vi "LoadGainCorrectionImages.vi"(8 "Pixel calibration":T1, 10 "MeasureConfig":T3={"Bead locations"=[{"X"=0, "Y"=0}], "ROI"=200, "Experiment base path"=path "", "Image output subdir"="images", "Output mode"=enum."None", "Traces output subdir"="traces", "QTrk Settings"={"Image width"=150, "Image height"=150, "Number of threads (CPU based)"=-1, "CUDA Device"=-2, "COM Background correction factor"=0.0, "ZLUT MinRadius"=8.0, "ZLUT Radial sample density"=5.0, "ZLUT Angular sample density"=2.0, "ZLUT ROI Coverage"=0.7, "QI Iterations"=1, "QI MinRadius"=2.0, "QI Radial sample density"=5.0, "QI Angular sample density"=2.0, "QI ROI Coverage"=0.7, "QI Angular Step \nIteration Factor"=0.8, "XCOR Profile Length"=1, "XCOR Profile Width"=128, "XCOR Iterations"=32, "Gaussian 2D Fit Iterations"=2, "Gaussian 2D Sigma (pixels)"=3.0, "Downsample"=0}, "Tracking Config"={"Number of steps"=0, "ZLUT stepsize (um)"=0.0, "Z correction factor"=0.0, "Start piezo Z (um)"=0.0, "Pixel size (nm)"=0.0, "2D Localization Type"=enum."Quadrant Interpolation", "Z Command (None)"=enum."Nothing", "Z Piezo scale"=FALSE, "ZLUT Building\nimages per frame"=1}, "Experiment Name"="", "Program"={"Commands"=[], "Motor Axis accuracy conditions"={"Magnet Z"=0.0, "Magnet rotation"=0.0, "Camera"={"X"=0.0, "Y"=0.0}, "Piezo XY"={"X"=0.0, "Y"=0.0}, "Piezo Z"=0.0, "Coil XY"={"X"=0.0, "Y"=0.0}}, "Axis flags"={"Magnet Z"=FALSE, "Magnet rotation"=FALSE, "Camera"={"X"=FALSE, "Y"=FALSE}, "Piezo XY"={"X"=FALSE, "Y"=FALSE}, "Piezo Z"=FALSE, "Coil XY"={"X"=FALSE, "Y"=FALSE}}}, "ZLUT"=[], "Camera settings"={"Framerate (Hz)"=60, "Exposure time (us)"=5000, "Image size"={"Width"=1280, "Height"=1024}, "Number of buffers"=30}, "Experiment Script"="", "Max frames in memory"=10000, "Save traces as binary"=FALSE, "Pixel Calibration Gain Image"="camera_calib_gain.bin", "Pixel Calibration Offset Image"="camera_calib_offset.bin", "Use pixel calibration images"=FALSE, "Internal camera settings"="", "Trace write interval"=100} {"QTrk Settings"."QI ROI Coverage" format="%_2g"; "QTrk Settings"."QI MinRadius" format="%.2f"; "QTrk Settings"."QI Angular sample density" format="%.3f"; "QTrk Settings"."QI Radial sample density" format="%.2f"; "QTrk Settings"."ZLUT Radial sample density" format="%.2f"; "QTrk Settings"."ZLUT MinRadius" format="%.2f"}, 11 "QTrk Instance in":T17) -> (0 "Pixel calibration(out)":T1, 3 "QTrk Instance out":T17)   [LabVIEW 2011]
uses:
  qtrk/QTrkLVBinding/QTrkInstance.ctl
  Typedefs/MeasureConfigType.ctl
  Typedefs/MeasureConfigOutputMode.ctl
  qtrk/QTrkLVBinding/QTrkSettings.ctl
  Typedefs/TrackingConfigType.ctl
  qtrk/QTrkLVBinding/QTrkLocalizationType.ctl
  qtrk/QTrkLVBinding/QTrkZCommandType.ctl
  ExperimentProgram/ExperimentProgramType.ctl
  ExperimentProgram/ExProgCommandType.ctl
  ExperimentProgram/ExProgCommandEnumType.ctl
  Motors/MotorAxisEnum.ctl
  Motors/MotorPosType.ctl
  Typedefs/XYf.ctl
  Motors/MotorPosFlagsType.ctl
  Camera/GenericCameraConfigType.ctl
  Camera/PixelCalibrationDataType.ctl
  <vilib>/vision/Image Controls.llb/IMAQ Image.ctl
panel:
  # "(used for commands with string parameters)"
  # "-2: Use all devices\n-1: Use best device"
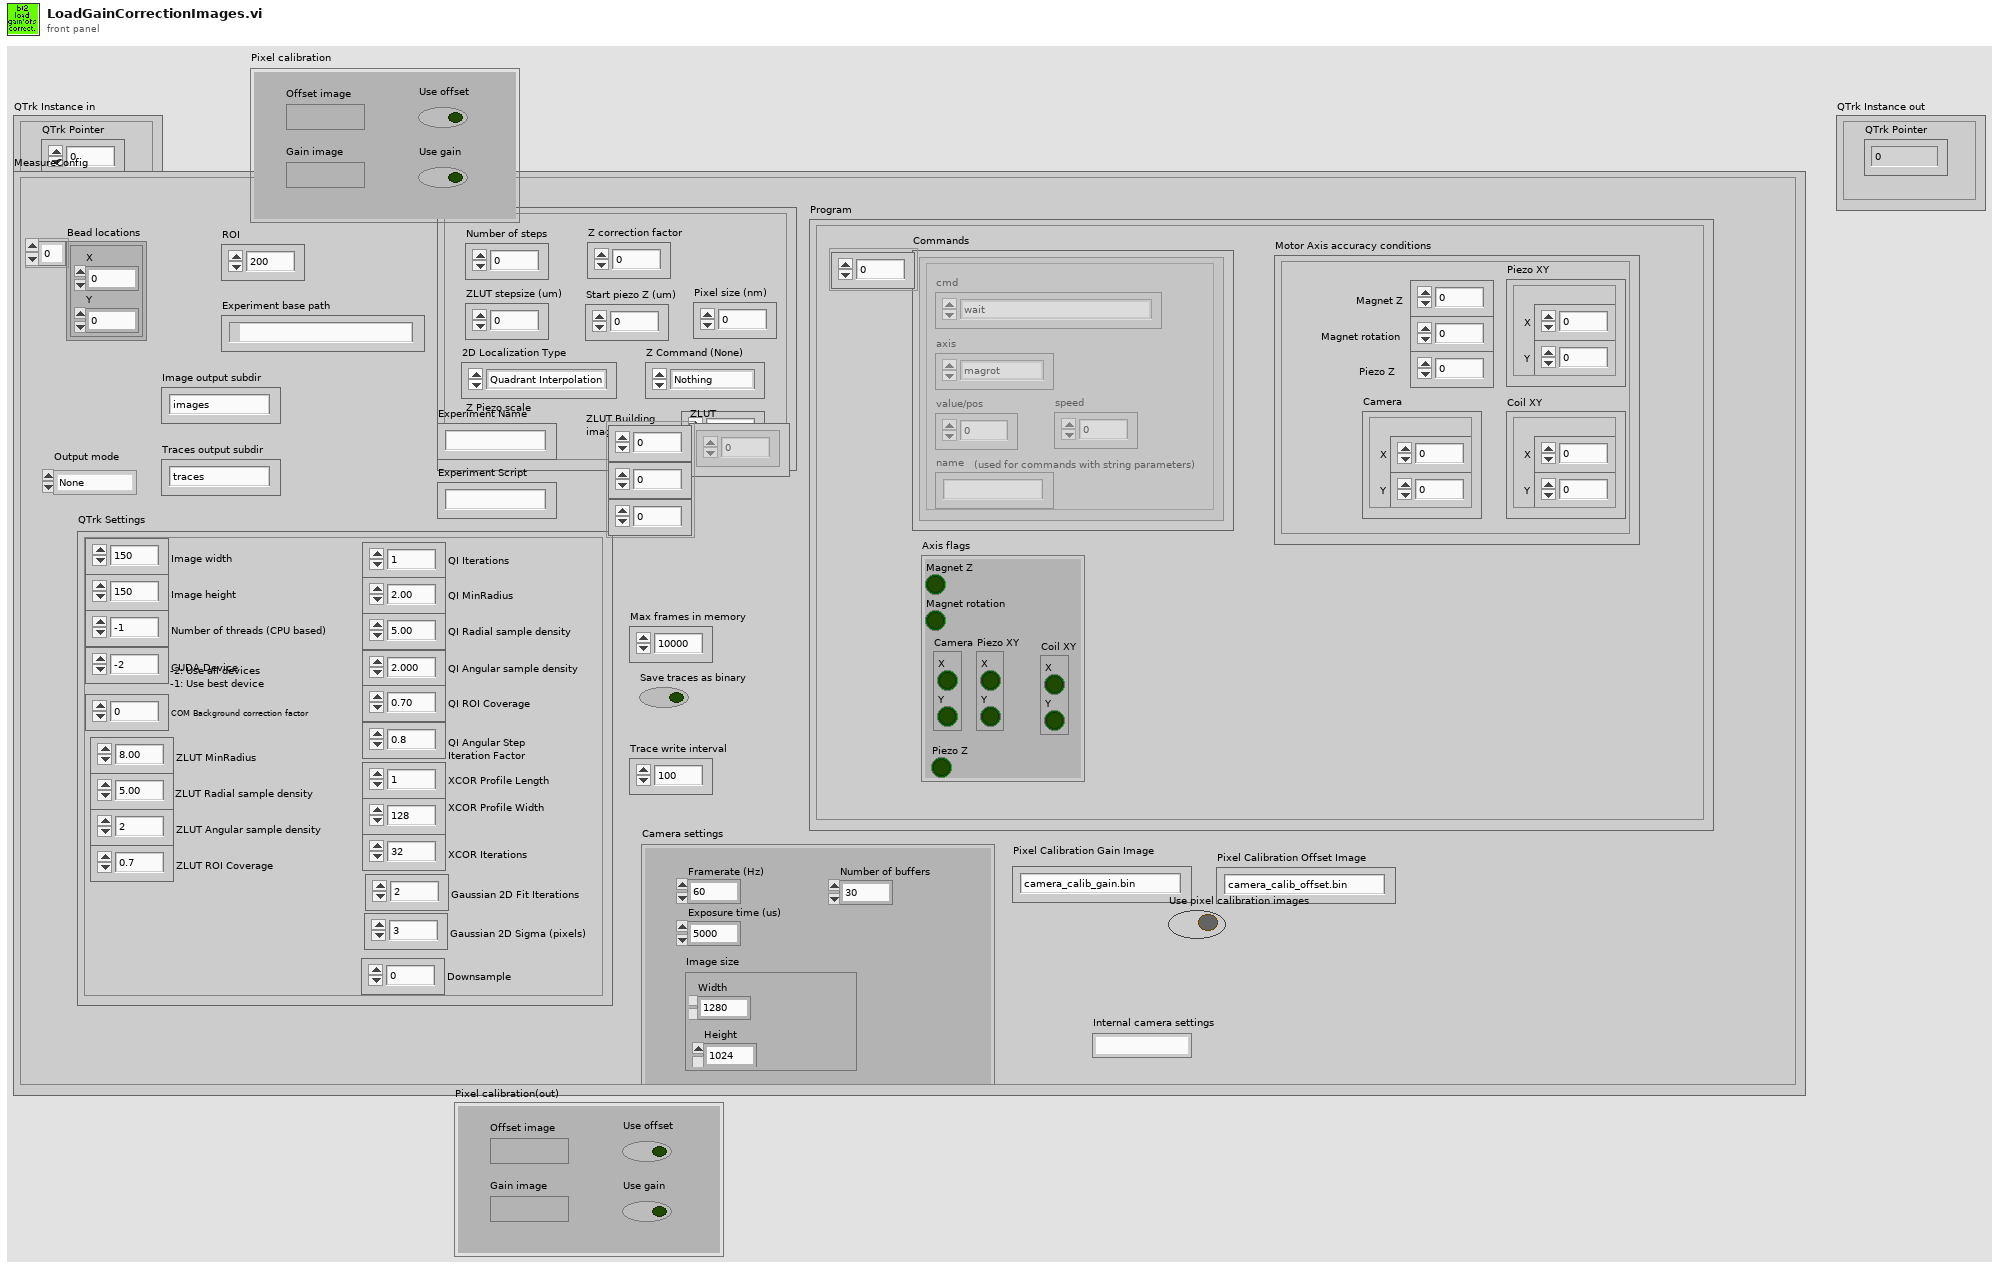
[diagram p1: front panel]
types:
  T1 = typedef "PixelCalibrationDataType.ctl" = cluster{"Offset image":T2, "Gain image":T2, "Use offset":bool, "Use gain":bool}
  T2 = typedef "IMAQ Image.ctl" = refnum<image>
  T3 = typedef "MeasureConfigType.ctl" = cluster{"Bead locations":cluster{"X":i32, "Y":i32}[], "ROI":i32, "Experiment base path":path, "Image output subdir":string, "Output mode":T4, "Traces output subdir":string, "QTrk Settings":T5, "Tracking Config":T6, "Experiment Name":string, "Program":T9, "ZLUT":sgl[][][], "Camera settings":T16, "Experiment Script":string, "Max frames in memory":i32, "Save traces as binary":bool, "Pixel Calibration Gain Image":string, "Pixel Calibration Offset Image":string, "Use pixel calibration images":bool, "Internal camera settings":string, "Trace write interval":i32}
  T4 = typedef "MeasureConfigOutputMode.ctl" = enum16{"None", "Track", "SaveImages"}
  T5 = typedef "QTrkSettings.ctl" = cluster{"Image width":i32, "Image height":i32, "Number of threads (CPU based)":i32, "CUDA Device":i32, "COM Background correction factor":sgl, "ZLUT MinRadius":sgl, "ZLUT Radial sample density":sgl, "ZLUT Angular sample density":sgl, "ZLUT ROI Coverage":sgl, "QI Iterations":i32, "QI MinRadius":sgl, "QI Radial sample density":sgl, "QI Angular sample density":sgl, "QI ROI Coverage":sgl, "QI Angular Step \nIteration Factor":sgl, "XCOR Profile Length":i32, "XCOR Profile Width":i32, "XCOR Iterations":i32, "Gaussian 2D Fit Iterations":i32, "Gaussian 2D Sigma (pixels)":sgl, "Downsample":i32}
  T6 = typedef "TrackingConfigType.ctl" = cluster{"Number of steps":i32, "ZLUT stepsize (um)":sgl, "Z correction factor":sgl, "Start piezo Z (um)":sgl, "Pixel size (nm)":sgl, "2D Localization Type":T7, "Z Command (None)":T8, "Z Piezo scale":bool, "ZLUT Building\nimages per frame":i32}
  T7 = typedef "QTrkLocalizationType.ctl" = enum16{"Center-of-Mass", "1D Cross-Correlation", "Quadrant Interpolation", "Gaussian 2D MLE", "QI + ZLUTAlign", "ZLUTAlign", "QI + FourierLUT"}
  T8 = typedef "QTrkZCommandType.ctl" = enum16{"Nothing", "ComputeZ", "BuildRadialZLUT", "BuildImageZLUT", "RadialZLUT+ImageZLUT"}
  T9 = typedef "ExperimentProgramType.ctl" = cluster{"Commands":T10[], "Motor Axis accuracy conditions":T13, "Axis flags":T15}
  T10 = typedef "ExProgCommandType.ctl" = cluster{"cmd":T11, "axis":T12, "value/pos":dbl, "speed":dbl, "name":string}
  T11 = typedef "ExProgCommandEnumType.ctl" = enum16{"wait", "move", "acquire", "idle", "rmove", "when", "section", "stop"}
  T12 = typedef "MotorAxisEnum.ctl" = enum16{"no axis", "magrot", "magpos", "px", "py", "pz", "camx", "camy"}
  T13 = typedef "MotorPosType.ctl" = cluster{"Magnet Z":dbl, "Magnet rotation":dbl, "Camera":T14, "Piezo XY":T14, "Piezo Z":dbl, "Coil XY":T14}
  T14 = typedef "XYf.ctl" = cluster{"X":sgl, "Y":sgl}
  T15 = typedef "MotorPosFlagsType.ctl" = cluster{"Magnet Z":bool, "Magnet rotation":bool, "Camera":cluster{"X":bool, "Y":bool}, "Piezo XY":cluster{"X":bool, "Y":bool}, "Piezo Z":bool, "Coil XY":cluster{"X":bool, "Y":bool}}
  T16 = typedef "GenericCameraConfigType.ctl" = cluster{"Framerate (Hz)":i32, "Exposure time (us)":i32, "Image size":cluster{"Width":i32, "Height":i32}, "Number of buffers":i32}
  T17 = typedef "QTrkInstance.ctl" = cluster{"QTrk Pointer":u64}
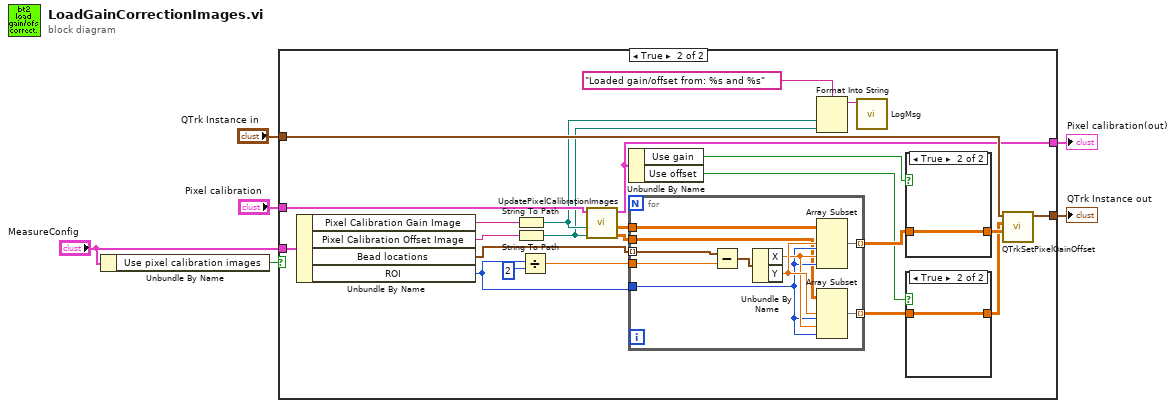
[diagram p0: block diagram]
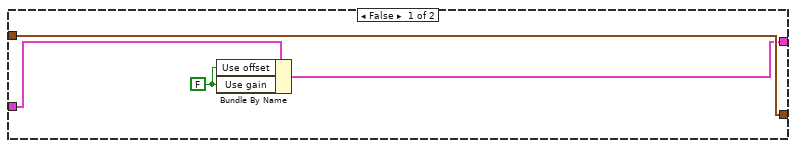
[diagram p2: hidden frame]
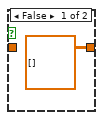
[diagram p3: hidden frame]
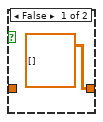
[diagram p4: hidden frame]
diagram:
  n1 = Unbundle By Name("MeasureConfig") -> ("Use pixel calibration images"=w4:bool)
  n2 = case shown="True" w4 {
    tunnel: "QTrk Instance in" -> [w10 w33]
    tunnel: [w10 w32] -> w6
    tunnel: "MeasureConfig" -> [_ w31]
    tunnel: [w8 w14] -> w2
    tunnel: "Pixel calibration" -> [w9 w13]
    frame False {
      w7 = FALSE ("Use offset")
      n3 = Bundle By Name(cluster=w9, "Use offset"=w7, "Use gain"=w7) -> (w8:T1)
    }
    frame True {
      n4 = Unbundle By Name(w31) -> ("Pixel Calibration Gain Image"=w30:string, "Pixel Calibration Offset Image"=w29:string, "Bead locations"=w26:cluster{"X":i32, "Y":i32}[], "ROI"=w23:i32)
      n5 = String To Path(string=w30) -> (path=w12:path)
      n6 = String To Path(string=w29) -> (path=w11:path)
      n7 = Divide(x=w23, y=2) -> (x/y=w24:dbl)
      n8 = call "UpdatePixelCalibrationImages.vi"("Pixel Calibration Offset Image"=w11, "Pixel Calibration Gain Image"=w12, "Pixel calibration"=w13) -> ("Offset"=w19:sgl[][], "Gain"=w20:sgl[][], "Pixel calibration"=w14:T1)  [unwired: 6 in]
      n9 = Unbundle By Name(w14) -> ("Use gain"=w21:bool, "Use offset"=w17:bool)
      n10 = for {
        tunnel: w26 -> [w46] mode=indexing
        tunnel: w20 -> [w47]
        tunnel: w24 -> [w45]
        tunnel: w23 -> [w40]
        tunnel: [w43] -> w22 mode=indexing
        tunnel: w19 -> [w39]
        tunnel: [w38] -> w16 mode=indexing
        n11 = Subtract(x=w46, y=w45) -> (x-y=w44:cluster{"X":dbl, "Y":dbl})
        n12 = Unbundle By Name(w44) -> ("X"=w41:dbl, "Y"=w42:dbl)
        n13 = Array Subset(array=w47, index (row)=w42, length (row)=w40, index (col)=w41, length (col)=w40) -> (w43:sgl[][])
        n14 = Array Subset(array=w39, index (row)=w42, length (row)=w40, index (col)=w41, length (col)=w40) -> (w38:sgl[][])
      }
      n15 = Format Into String(format string="Loaded gain/offset from: %s and %s", w12, w11) -> (resulting string=w27:string)  [unwired: 2 in, 1 out]
      n16 = call "LogMsg.vi"("msg"=w27) -> ()  [unwired: 11 in]
      n17 = case shown="True" w21 {
        tunnel: w22 -> [_ w37]
        tunnel: [sgl[][][] [] w37] -> w18
        frame False {
        }
        frame True {
        }
      }
      n18 = case shown="True" w17 {
        tunnel: w16 -> [_ w35]
        tunnel: [sgl[][][] [] w35] -> w15
        frame False {
        }
        frame True {
        }
      }
      n19 = call "QTrkSetPixelGainOffset.vi"("Gain"=w18, "Offset"=w15, "QTrk Instance"=w33) -> ("QTrk Instance"=w32:T17)  [unwired: 7 in, 1 out]
    }
  }
  "QTrk Instance out" <- w6
  "Pixel calibration(out)" <- w2
